vi "MyInterfaceMethod.vi"(0 "reference in":refnum<class "MyClass5.lvclass">, 1 "MyParameter":dbl, 5 "error in (no error)":errorcluster) -> (14 "reference out":refnum<class "MyClass5.lvclass">, 19 "error out":errorcluster)   [LabVIEW 2020, in "MyClass5.lvclass"]
uses:
  MyClass5.lvclass
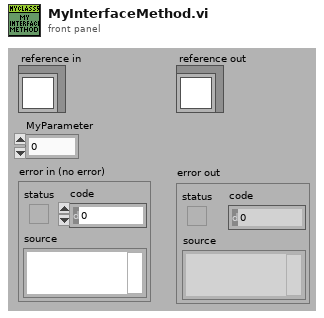
[diagram p1: front panel]
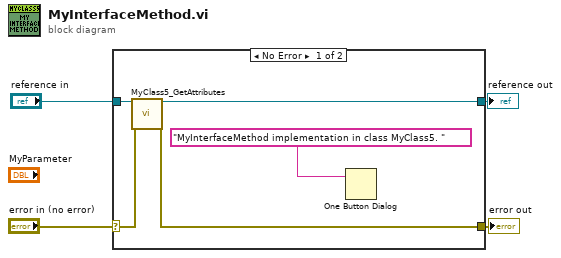
[diagram p0: block diagram]
diagram:
  n1 = case shown="No Error" "error in (no error)" {
    selector: "error in (no error)" -> [w9 w11]
    tunnel: [w8 w11] -> w3
    tunnel: [w7 w10] -> w1
    tunnel: "reference in" -> [w6 w10]
    frame No Error {
      n2 = call "MyClass5_GetAttributes.vi"("reference in"=w6, "error in (no error)"=w9) -> ("reference out"=w7:refnum<class "MyClass5.lvclass">, "error out"=w8:errorcluster)  [unwired: 14 in, 2 out]
      n3 = One Button Dialog(message="MyInterfaceMethod implementation in class MyClass5. ") -> ()  [unwired: 1 in, 1 out]
    }
    frame Error {
    }
  }
  "error out" <- w3
  "reference out" <- w1
